vi "I16 tif save.vi"() -> ()   [LabVIEW 2015]
panel:
  out "Image Pixels (I16)":i16[][](array[numeric])
  out "Image":T1(plugin-control)
  in  "output":i16[][](array[numeric])=array512x512[262144 elements]
  in  "Path":path=path "C:/Users/TVS001/Desktop/DATA/20180207/13-zz-gcamp" caption="Images Folder"
  in  "File Name":string
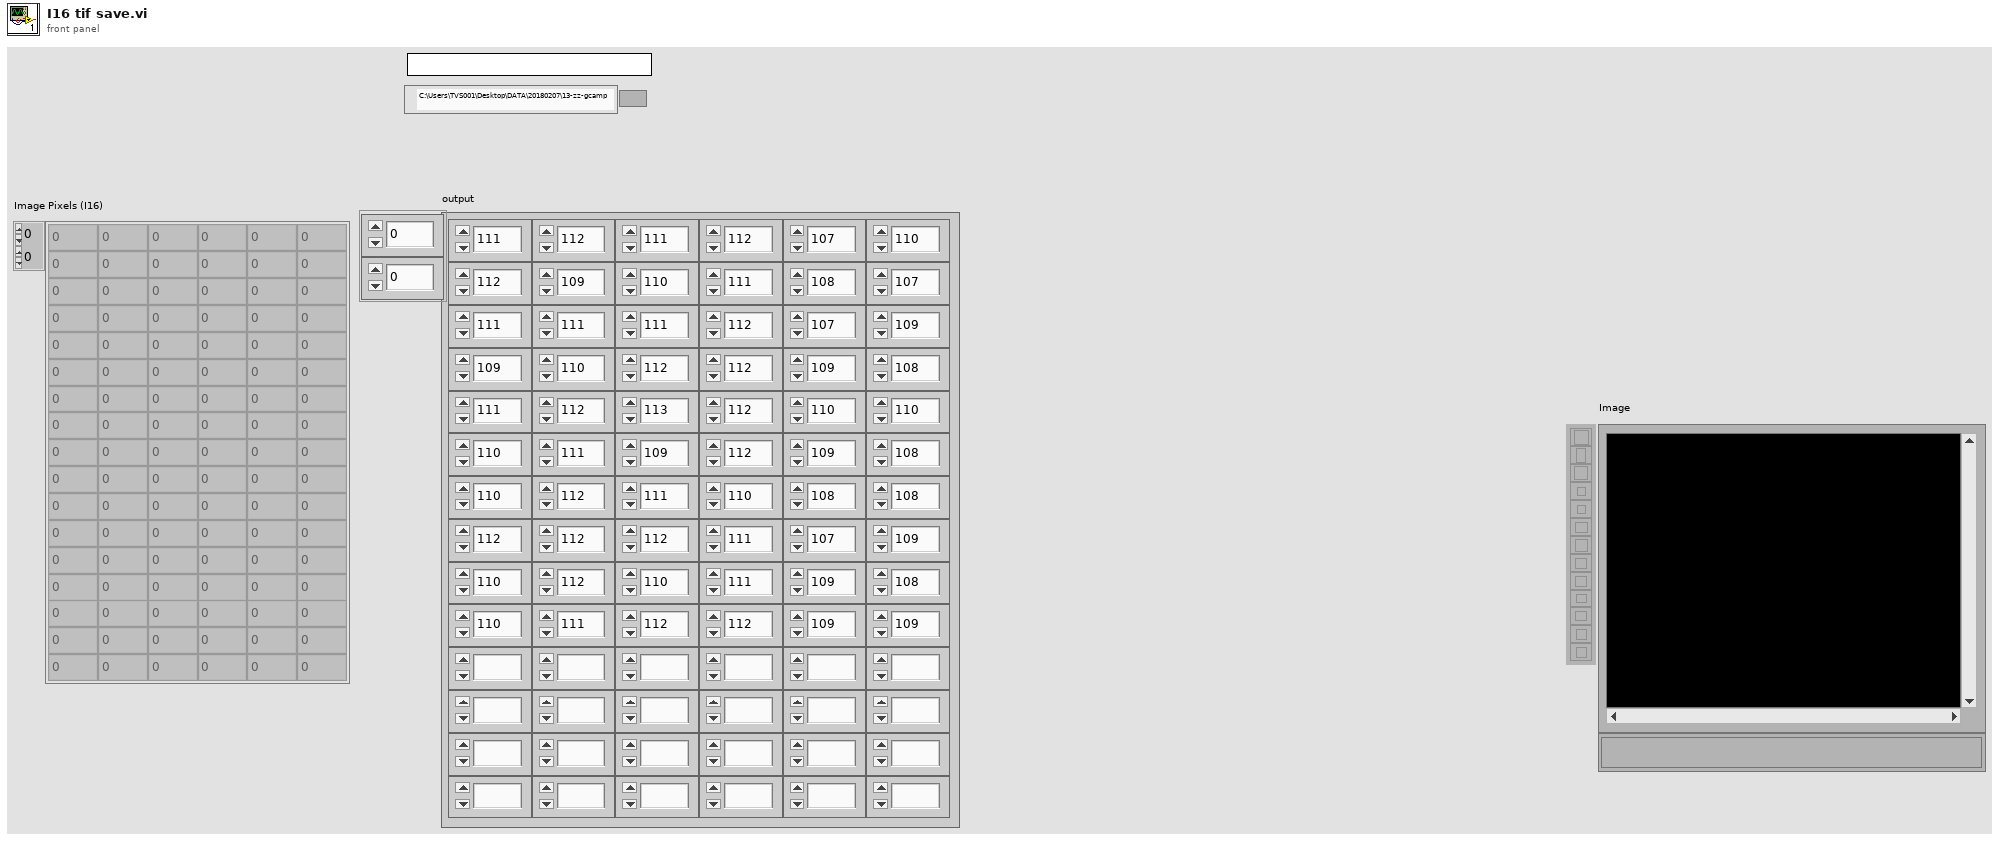
[diagram p1: front panel]
types:
  T1 = typedef "IMAQ Image.ctl" = refnum<image>
  T2 = typedef "Image Type" = u32
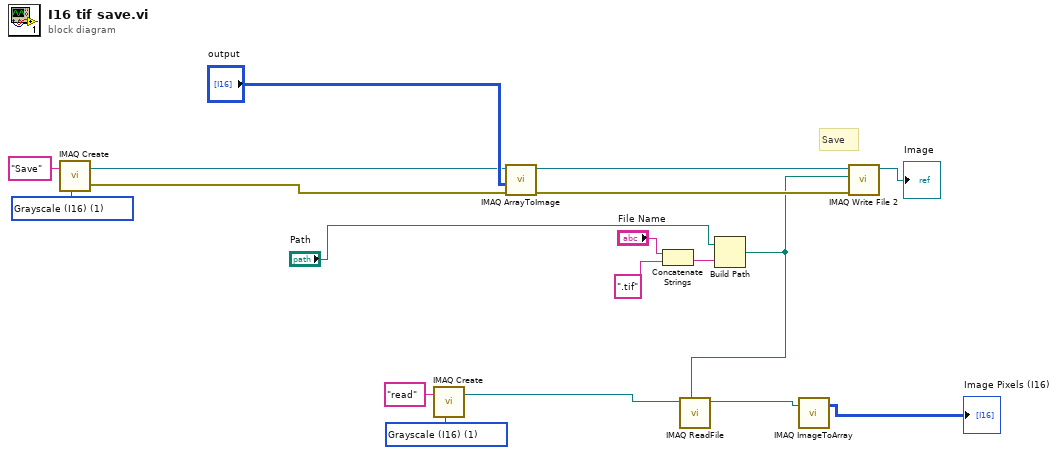
[diagram p0: block diagram]
diagram:
  w5 = T2 1 items=["Grayscale (U8)", "Grayscale (I16)", "Grayscale (SGL)", "Complex (CSG)", "RGB (U32)", "HSL (U32)", "RGB (U64)", "Grayscale (U16)"] ("Image Type")
  w12 = T2 1 items=["Grayscale (U8)", "Grayscale (I16)", "Grayscale (SGL)", "Complex (CSG)", "RGB (U32)", "HSL (U32)", "RGB (U64)", "Grayscale (U16)"] ("Image Type")
  # "Save"
  n1 = call "IMAQ Create"("Image Name"="Save", "Image Type"=w12) -> ("New Image"=w10:T1, "error out"=w9:errorcluster)  [unwired: 3 in]
  n2 = call "IMAQ Create"("Image Name"="read", "Image Type"=w5) -> ("New Image"=w2:T1)  [unwired: 3 in, 1 out]
  n3 = call "IMAQ ArrayToImage"("error in (no error)"=w9, "Image Pixels (I16)"="output", "Image"=w10) -> ("error out"=w8:errorcluster, "Image Out"=w14:T1)  [unwired: 7 in]
  n4 = Concatenate Strings("File Name", ".tif" ("字符串")) -> (w16:string)
  n5 = Build Path(base path="Path", name or relative path=w16) -> (appended path=w1:path)
  n6 = call "IMAQ ReadFile"("File Path"=w1, "Image"=w2) -> ("Image Out"=w4:T1)  [unwired: 5 in, 4 out]
  n7 = call "IMAQ ImageToArray"("Image"=w4) -> ("Image Pixels (I16)"=→"Image Pixels (I16)":i16[][])  [unwired: 3 in, 4 out]
  n8 = call-poly "IMAQ Write File 2"("error in (no error)"=w8, "File Path"=w1, "Image"=w14) -> ("Image Out (duplicate)"=→"Image":T1)  [unwired: 7 in, 1 out]
